vi "Initialize.vi"(8 "error in (no error)":errorcluster, 9 "Reset? (T: Yes)":bool=TRUE, 11 "VISA Tegam4040":refnum<visa-resource-name>) -> (0 "error out":errorcluster, 3 "VISA resource name out":refnum<visa-resource-name>)   [LabVIEW 2010, in "Tegam4040.lvlib"]
doc: "Establishes communication with the instrument and optionally performs an instrument reset. It also places the instrument in a default state needed for other instrument driver operations. Therefore, call this VI before calling other instrument driver VIs for this instrument. Generally, you need to call the <B>Initialize VI</B> only once at the beginning of an application."
uses:
  Tegam4040.lvlib
  <vilib>/Utility/error.llb/DialogType.ctl
panel:
  # "© 2007 Tegam INC.  ALL RIGHTS RESERVED."
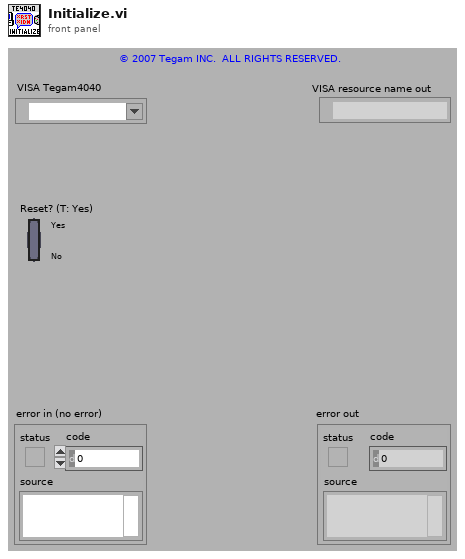
[diagram p1: front panel]
types:
  T1 = typedef "DialogType.ctl" = u16
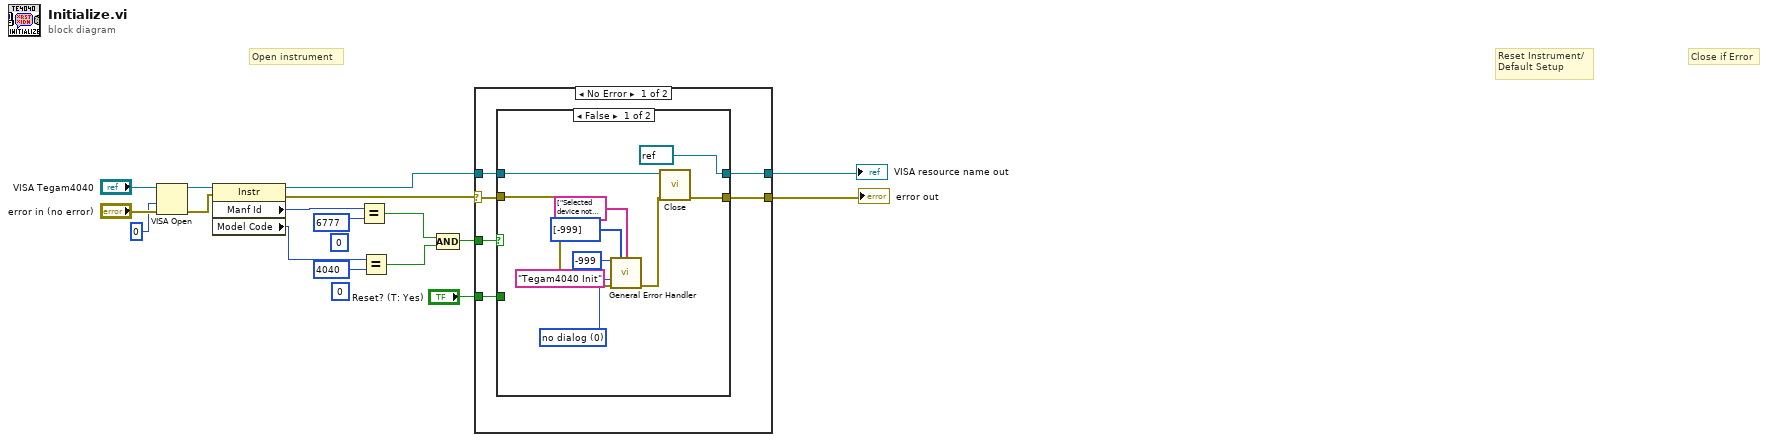
[diagram p0: block diagram]
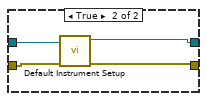
[diagram p3: hidden frame]
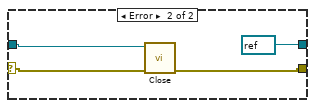
[diagram p4: hidden frame]
diagram:
  (unwired) u16 0 ("y")
  (unwired) u16 0 ("y")
  # "Close if Error"
  # "Reset Instrument/\nDefault Setup"
  # "Open instrument"
  n1 = VISA Open(access mode=u32 0, error in (no error)="error in (no error)", VISA resource name="VISA Tegam4040") -> (VISA resource name=w14:refnum<visa-resource-name>, error out=w13:errorcluster)  [unwired: 2 in]
  n2 = property class="Instr"(reference=w14, error in=w13) -> (reference out=w7:refnum<visa-resource-name>, error out=w6:errorcluster, "Manf Id"=w12:u16, "Model Code"=w11:u16)
  n3 = Equal?(x=w12, y=u16 6777) -> (x = y?=w10:bool)
  n4 = Equal?(x=w11, y=u16 4040) -> (x = y?=w9:bool)
  n5 = Compound Arithmetic op=AND(w10, w9) -> (w8:bool)
  n6 = case shown="No Error" w6 {
    selector: w6 -> [w19 w46]
    tunnel: w8 -> [w23 _]
    tunnel: [w22 w45] -> w4
    tunnel: w7 -> [w21 w48]
    tunnel: [w20 refnum<visa-resource-name> refnum ("VISA resource name out")] -> w5
    tunnel: "Reset? (T: Yes)" -> [w18 _]
    frame No Error {
      n7 = case shown="False" w23 {
        tunnel: w19 -> [w33 w35]
        tunnel: [w25 w34] -> w22
        tunnel: w21 -> [w27 w37]
        tunnel: [refnum<visa-resource-name> refnum ("VISA Tegam4040") w36] -> w20
        tunnel: w18 -> [_ w38]
        frame False {
          w32 = T1 0 items=["no dialog", "OK message", "continue or stop message", "OK message + warnings", "continue/stop + warnings"] ("type of dialog (OK msg:1)")
          n8 = call <vilib>:"General Error Handler.vi"("[error code] (0)"=-999, "[user-defined codes]"=i32[] [-999], "[user-defined descriptions]"=string[] ["Selected device not found"], "[error source] (\" \")"="Tegam4040 Init" ("[error source] (\" \")"), "type of dialog (OK msg:1)"=w32, "error in (no error)"=w33) -> ("error out"=w26:errorcluster)  [unwired: 5 in, 4 out]
          n9 = call "Close.vi"("error in (no error)"=w26, "VISA Tegam4040"=w27) -> ("error out"=w25:errorcluster)  [unwired: 9 in]
        }
        frame True {
          n10 = case shown="False" w38 {
            tunnel: [w40 w42] -> w36
            tunnel: w37 -> [w40 w44]
            tunnel: w35 -> [w39 w43]
            tunnel: [w39 w41] -> w34
            frame False {
            }
            frame True {
              n11 = call "Default Instrument Setup.vi"("error in (no error)"=w43, "VISA resource name"=w44) -> ("error out"=w41:errorcluster, "VISA resource name out"=w42:refnum<visa-resource-name>)  [unwired: 8 in]
            }
          }
        }
      }
    }
    frame Error {
      n12 = call "Close.vi"("error in (no error)"=w46, "VISA Tegam4040"=w48) -> ("error out"=w45:errorcluster)  [unwired: 9 in]
    }
  }
  "VISA resource name out" <- w5
  "error out" <- w4
